vi "Wait on acq completed.vi"() -> (3 "Timed out waiting":bool)   [LabVIEW 2020]
uses:
  Global Variables/General Globals.vi
panel:
  out "Acquisition completed":bool
  out "Elapsed Time (s)":dbl
  out "Final Time (s)":dbl format="%#_2f"
  out "Loop iteration":i32
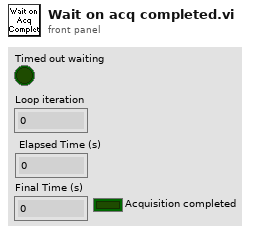
[diagram p1: front panel]
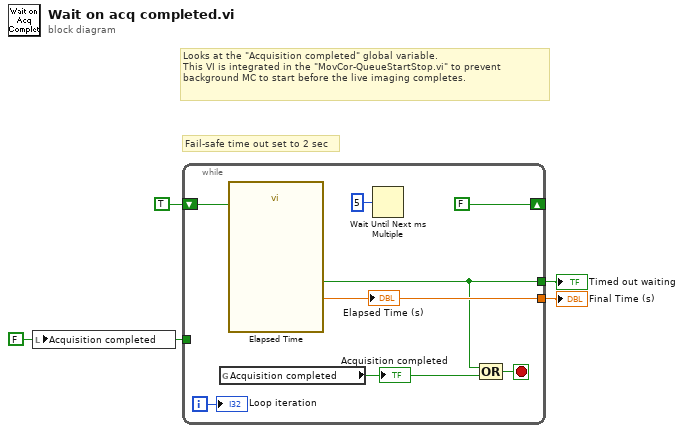
[diagram p0: block diagram]
diagram:
  w1 = FALSE ("Acquisition completed")
  # "Looks at the \"Acquisition completed\" global variable. \nThis VI is integrated in the \"MovCor-QueueStartStop.vi\" to prevent background MC to start before the live imaging completes."
  # "Fail-safe time out set to 2 sec"
  n1 = local write "Acquisition completed"(w1) -> ()
  n2 = while {
    shift-right: [FALSE] -> _
    shift-left: TRUE -> [w11]
    tunnel: [w6] -> w4
    tunnel: [w8] -> w3
    tunnel: w1 -> [_]
    i -> [w9]
    stop <- w7 stop-if-true
    n3 = global read "General Globals.vi" "Acquisition completed"() -> (w5:bool)
    "Acquisition completed" <- w5
    n4 = call "Elapsed Time"("Reset"=w11) -> ("Elapsed Time (s)"=w8:dbl, "Time has Elapsed"=w6:bool)  [unwired: 11 in, 6 out]
    "Elapsed Time (s)" <- w8
    n5 = Wait Until Next ms Multiple(millisecond multiple=u32 5) -> ()  [unwired: 1 out]
    n6 = Compound Arithmetic op=OR(w6, w5) -> (w7:bool)
    "Loop iteration" <- w9
  }
  "Timed out waiting" <- w4
  "Final Time (s)" <- w3
